vi "getEdgeLength.vi"(11 "StationKeeping in":refnum<class "StationKeeping.lvclass">) -> (1 "Edge Length":dbl, 3 "StationKeeping out":refnum<class "StationKeeping.lvclass">)   [LabVIEW 2011, in "StationKeeping.lvclass"]
doc: "Returns the length of one edge of the station (helpful for giving the scale of the station, to know, for example, how big a pattern to use for sailing inside the station)."
uses:
  StationKeeping.lvclass
  StationKeeping.lvclass/StationKeeping.ctl
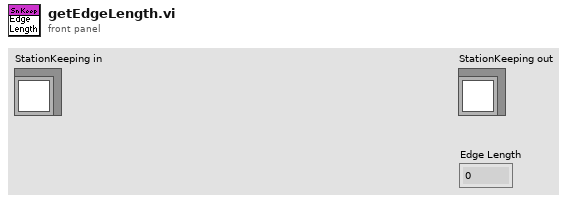
[diagram p1: front panel]
types:
  T1 = typedef "UTM Location.ctl" = cluster{"UTM Zone":dbl, "Hemisphere":enum16{"North", "South"}, "East":dbl, "North":dbl}
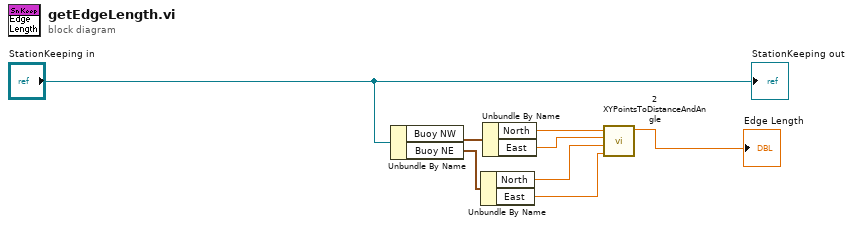
[diagram p0: block diagram]
diagram:
  n1 = Unbundle By Name("StationKeeping in") -> ("Buoy NW"=w7:T1, "Buoy NE"=w6:T1)
  n2 = Unbundle By Name(w6) -> ("North"=w3:dbl, "East"=w2:dbl)
  n3 = Unbundle By Name(w7) -> ("North"=w5:dbl, "East"=w4:dbl)
  n4 = call "2 XYPointsToDistanceAndAngle.vi"("East 2"=w2, "North 2"=w3, "East 1"=w4, "North 1"=w5) -> ("Distance"=→"Edge Length":dbl)  [unwired: 6 in, 1 out]
  "StationKeeping out" <- "StationKeeping in"
